vi "Main Config.vi"(8 "error in (no error)":errorcluster, 11 "Module_Refs":T1={"ModuleName"=enum."Controller", "Queue"=refnum, "user event"=refnum, "VI Refnum"=refnum, "ShowFP"=FALSE, "StatesTracking Enabled"=FALSE}) -> (0 "error out":errorcluster)   [LabVIEW 2021, in "Configuration.lvlib"]
doc: "Main Module Template of the architecture. Use this as a template to integrate new independent processes into your application."
uses:
  Configuration.lvlib
  Typedefs/Module References.ctl
  Typedefs/Enum_Module_Name.ctl
  Typedefs/Message.ctl
  Typedefs/SM Data.ctl
  Typedefs/App Cfg DVR.ctl
  Typedefs/Application Configuration.ctl
  Module Template/Typedefs/Config.ctl
  Core UI/Typedefs/Config.ctl
  Modules/Sound Manager/Typedefs/Config.ctl
  Typedefs/FGV Ref. Modules Function.ctl
  <vilib>/event_ctls.llb/usereventprio.ctl
  Architecture.lvlib
  Modules/Sound Manager/Sound Manager.lvlib
  Core UI/Core UI.lvlib
  Module Template/Module Template.lvlib
panel:
  in  "Stop App":bool
  out "Message":string
  in  "Stop Module":bool
  # "#Architecture\n\nPlace inside this box all visible data."
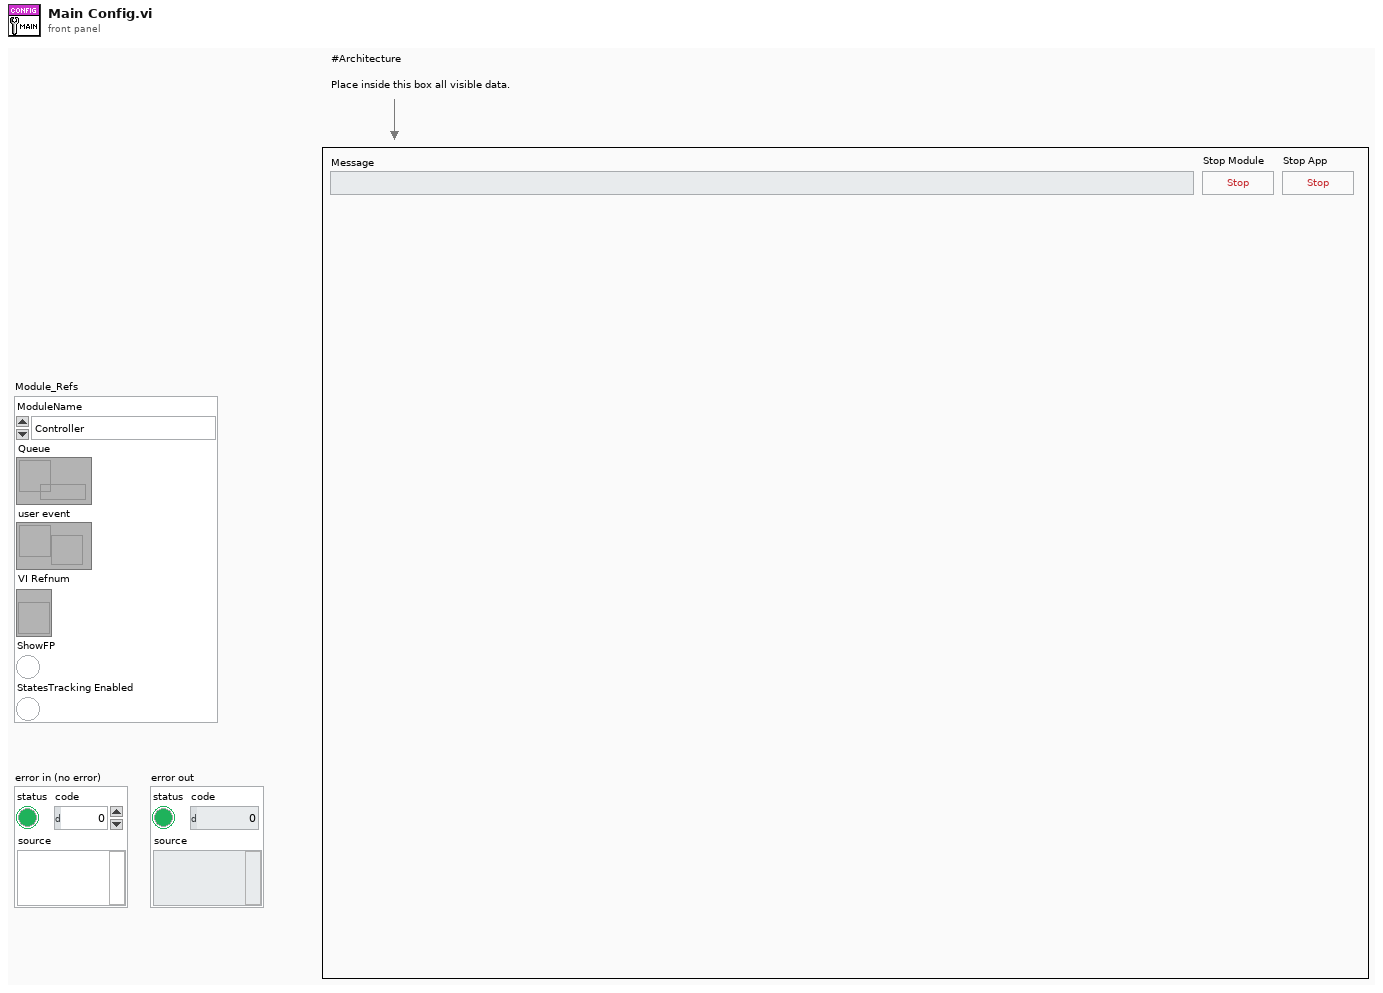
[diagram p1: front panel]
types:
  T1 = typedef "Architecture.lvlib/Module References.ctl" = cluster{"ModuleName":T2, "Queue":refnum<queue>, "user event":refnum<user-event>, "VI Refnum":refnum<vi>, "ShowFP":bool, "StatesTracking Enabled":bool}
  T2 = typedef "Configuration.lvlib/Enum_Module_Name.ctl" = enum16{"Configuration", "Error_Handler", "Log", "Database", "Controller", "UI Module", "Sound Manager"}
  T3 = typedef "Configuration.lvlib/SM Data.ctl" = cluster{"Module_Refs":T1, "Response Data":variant, "Config app":T4}
  T4 = typedef "Configuration.lvlib/App Cfg DVR.ctl" = refnum<data-value>
  T5 = enum32{"Invalid", "Standard", "Closed", "Hidden", "Minimized", "Maximized"}
  T6 = typedef "Error_Manager.lvlib/LogRotate.lvclass/LogData.ctl" = cluster{"error in":errorcluster, "replacements":string[], "Time Stamp":timestamp}
  T7 = typedef "Architecture.lvlib/FGV Ref. Modules Function.ctl" = enum16{"Init ", "Add Module", "Get Module", "Get All", "Add Asynchronous Run Ref", "Dispose"}
  T8 = typedef "usereventprio.ctl" = enum32{"high priority", "normal priority"}
  T9 = typedef "Configuration.lvlib/Application Configuration.ctl" = cluster{"Module Template Config":T10, "Core UI Config":T11, "Sound Manager Config":T12}
  T10 = typedef "Module Template.lvlib/Config.ctl" = cluster{"Module Enabled":bool}
  T11 = typedef "Core UI.lvlib/Config.ctl" = cluster{"Module Enabled":bool}
  T12 = typedef "Sound Manager.lvlib/Config.ctl" = cluster{"Sound Library Path":path, "dyn sounds path":path}
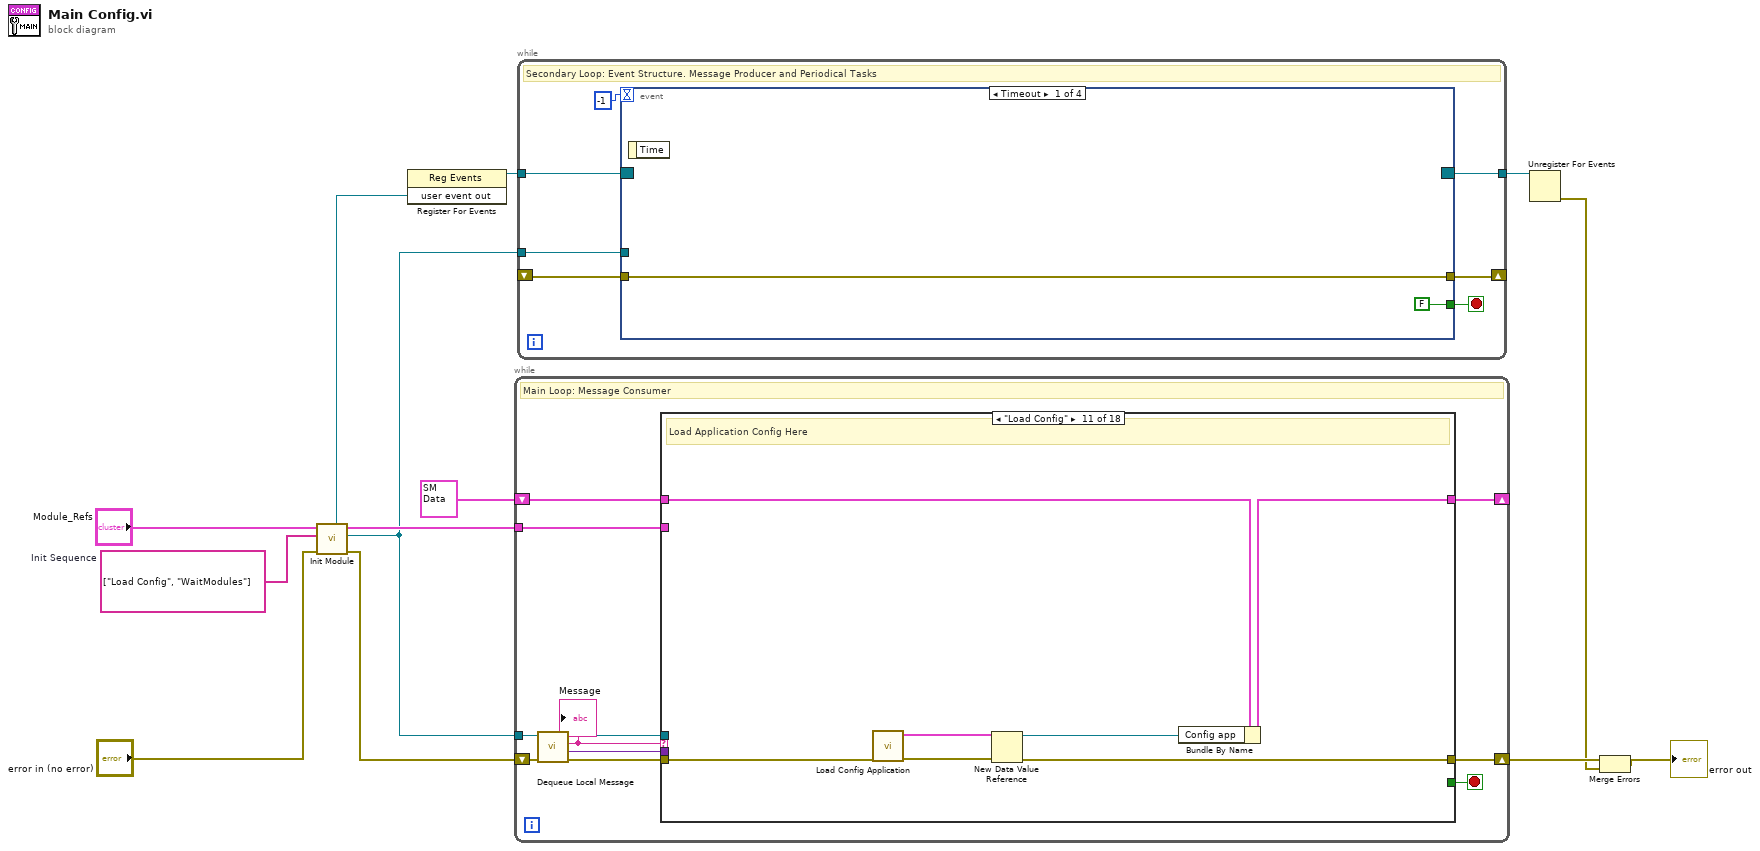
[diagram p0: block diagram]
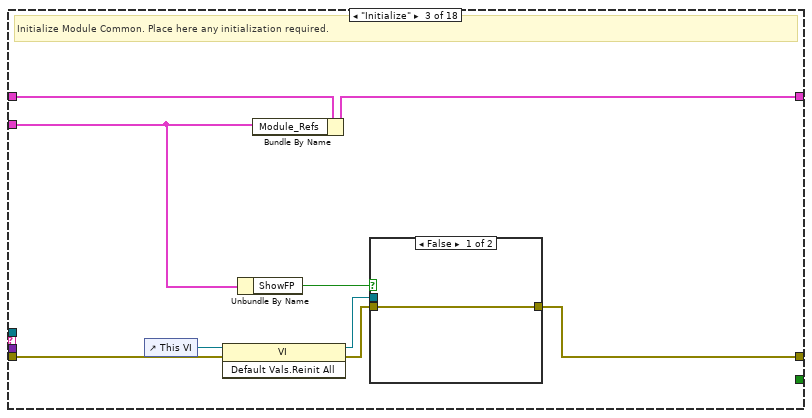
[diagram p4: hidden frame]
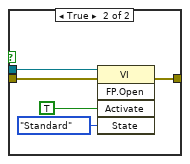
[diagram p5: hidden frame]
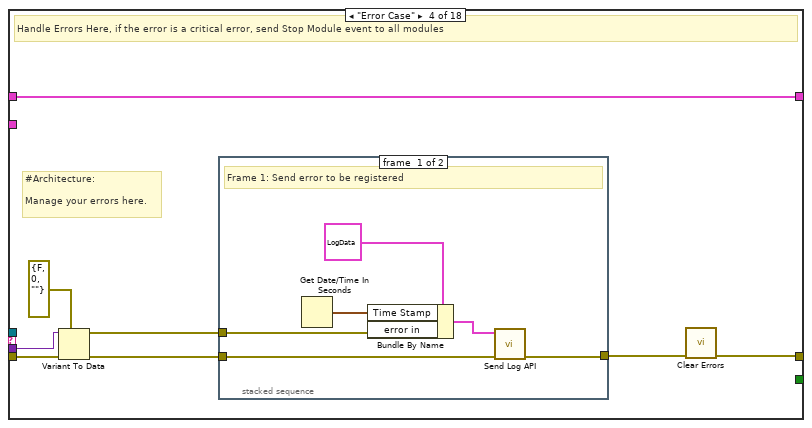
[diagram p6: hidden frame]
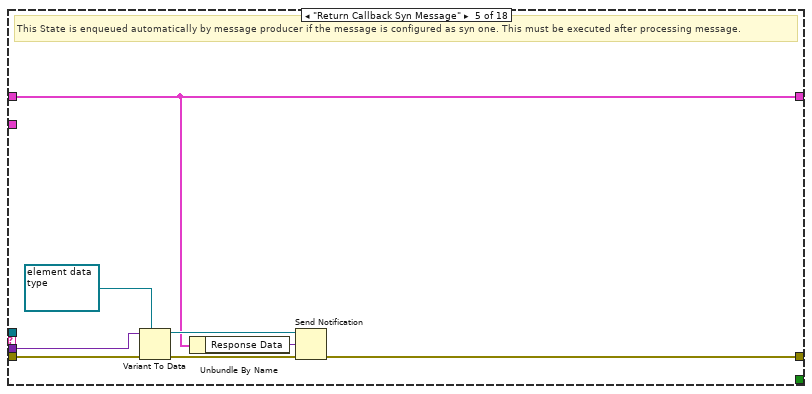
[diagram p9: hidden frame]
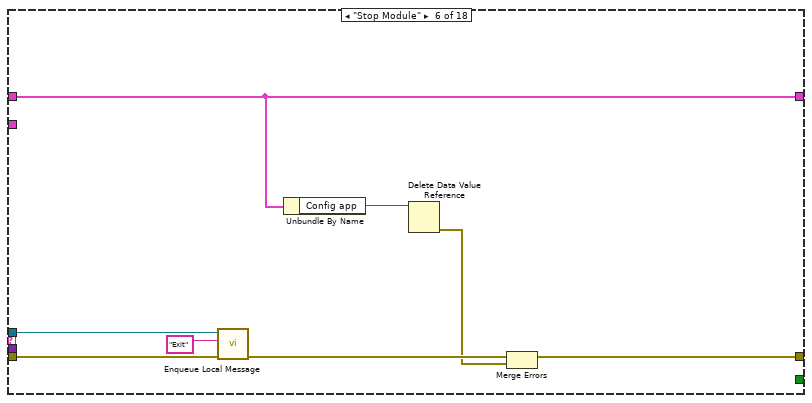
[diagram p10: hidden frame]
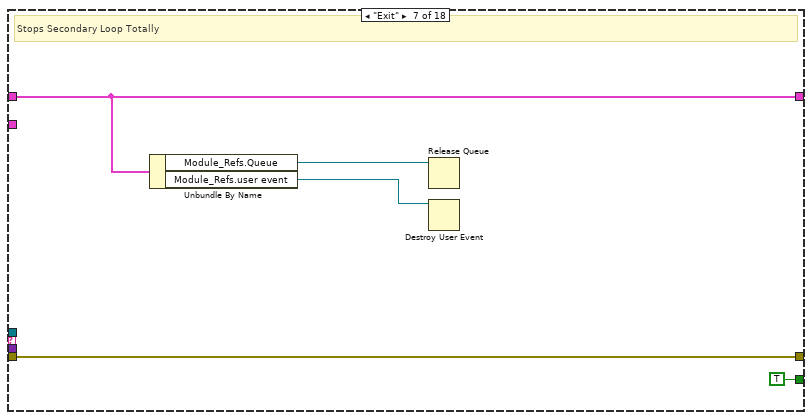
[diagram p11: hidden frame]
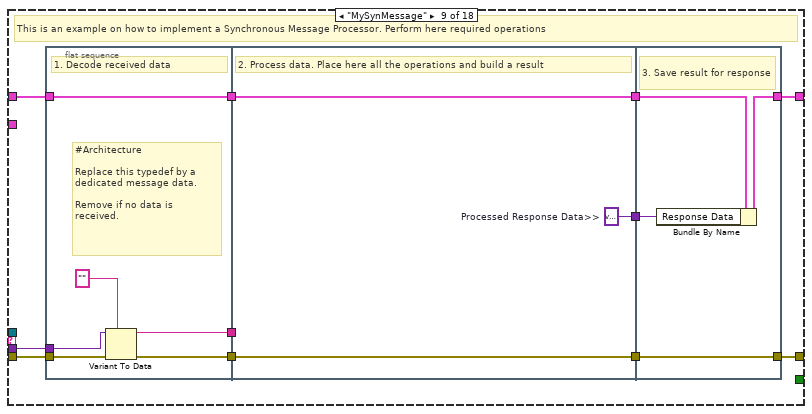
[diagram p13: hidden frame]
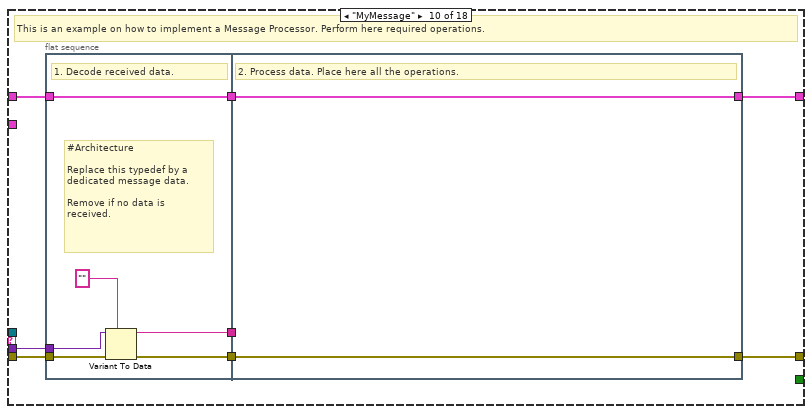
[diagram p14: hidden frame]
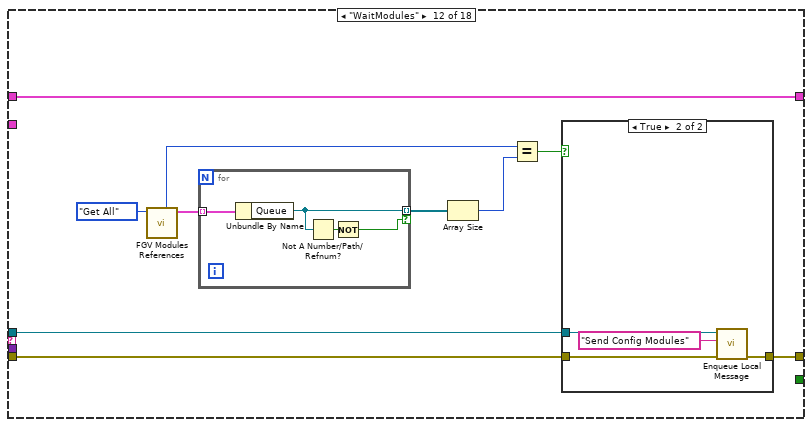
[diagram p15: hidden frame]
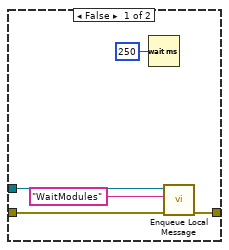
[diagram p16: hidden frame]
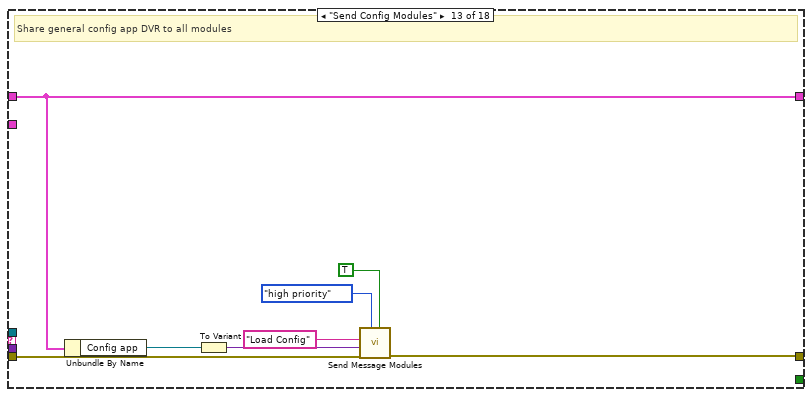
[diagram p17: hidden frame]
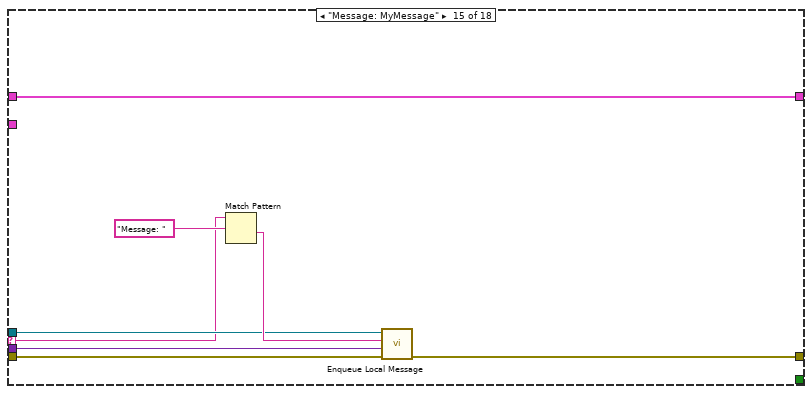
[diagram p19: hidden frame]
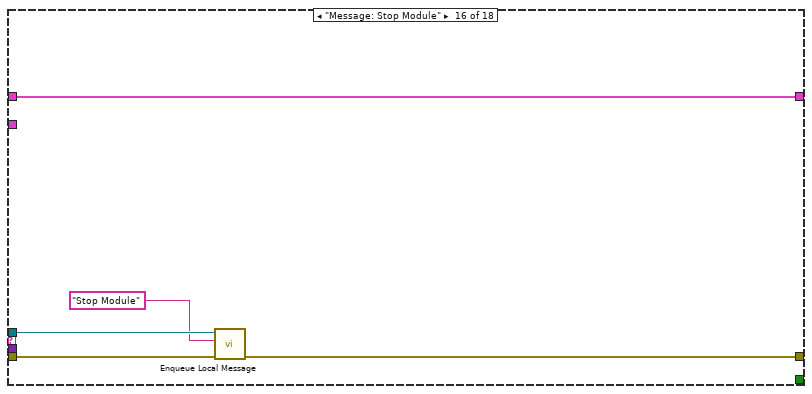
[diagram p20: hidden frame]
diagram:
  w11 = string[] ["Load Config", "WaitModules"]  # Init Sequence
  n1 = call "Init Module.vi"("error in (no error)"="error in (no error)", "Init Sequence"=w11, "Module Refs"="Module_Refs") -> ("error out"=w13:errorcluster, "queue out"=w2:refnum<queue>, "Module Refs Out"=w4:T1, "user event out"=w3:refnum<user-event>)  [unwired: 5 in]
  n2 = register-events(w3) -> (reference out=w10:refnum<event-registration>)  [unwired: 2 in, 1 out]
  n3 = while {
    shift-right: [w23] -> _
    shift-left: T3 {"Module_Refs"={"ModuleName"=enum."Controller", "Queue"=refnum, "user event"=refnum, "VI Refnum"=refnum, "ShowFP"=FALSE, "StatesTracking Enabled"=FALSE}, "Response Data"=variant, "Config app"=refnum} ("SM Data") -> [w24]
    shift-right: [w22] -> w8
    shift-left: w13 -> [w20]
    tunnel: w2 -> [w21]
    tunnel: w4 -> [w14]
    stop <- w15 stop-if-true
    # "Main Loop: Message Consumer"
    n4 = call "Dequeue Local Message.vi"("error in"=w20, "Msg queue in"=w21) -> ("error out"=w19:errorcluster, "Data"=w16:variant, "Message"=w17:string, "queue out"=w18:refnum<queue>)  [unwired: 6 in]
    "Message" <- w17
    n5 = case shown="\"Load Config\"" w17 {
      selector: w17 -> [_ _ _ _ _ _ _ _ _ _ _ _ _ _ w165 _ _ w188]
      tunnel: w24 -> [w26 w28 w37 w51 w63 w73 w80 w84 w95 w116 w131 w141 w157 w164 w172 w177 w179 w193]
      tunnel: [w26 w28 w35 w51 w63 w73 w80 w84 w94 w109 w127 w141 w157 w164 w172 w177 w179 w193] -> w23
      tunnel: w19 -> [w25 w27 w36 w50 w69 w77 w82 w83 w88 w112 w130 w134 w162 w163 w169 w176 w178 w192]
      tunnel: [w25 w27 w31 w44 w68 w72 w82 w83 w93 w115 w126 w133 w161 w163 w166 w175 w178 w182] -> w22
      tunnel: w18 -> [_ _ _ _ _ w75 _ _ _ _ _ w135 _ _ w167 w174 _ w189]
      tunnel: w16 -> [_ _ _ w49 w66 _ _ _ w87 w111 _ _ _ _ w168 _ _ w190]
      tunnel: [_ _ _ _ _ _ TRUE _ _ _ _ _ _ _ _ _ _ _] -> w15
      tunnel: w14 -> [_ _ w34 _ _ _ _ _ _ _ _ _ _ _ _ _ _ _]
      frame "--------State Machine Arquitechture Operations--------" {
      }
      frame "Idle", Default {
        # "Use this state to make iterations if required."
      }
      frame "Initialize" {
        # "Initialize Module Common. Place here any initialization required."
        n6 = control-ref of="This VI"() -> (w29:refnum<vi>)
        n7 = invoke class="VI" method="Default Vals.Reinit All"(reference=w29, error in=w36) -> (reference out=w32:refnum<vi>, error out=w33:errorcluster)  [unwired: 1 in, 1 out]
        n8 = Unbundle By Name(w34) -> ("ShowFP"=w30:bool)
        n9 = Bundle By Name(cluster=w37, "Module_Refs"=w34) -> (w35:T3)
        n10 = case shown="False" w30 {
          tunnel: w33 -> [w38 w43]
          tunnel: [w38 w42] -> w31
          tunnel: w32 -> [_ w41]
          frame False {
          }
          frame True {
            n11 = invoke class="VI" method="FP.Open"(reference=w41, error in=w43, "Activate"=TRUE ("Activate?"), "State"=T5."Standard") -> (error out=w42:errorcluster)  [unwired: 1 in, 4 out]
          }
        }
      }
      frame "Error Case" {
        # "#Architecture: \n\nManage your errors here."
        # "Handle Errors Here, if the error is a critical error, send Stop Module event to all modules"
        n12 = Variant To Data(error in=w50, type=errorcluster {"status"=FALSE, "code"=0, "source"=""} ("error constant"), Variant=w49) -> (data=w45:errorcluster, error out=w47:errorcluster)
        n13 = stacked-sequence {
          tunnel: w47 -> [w57 w59]
          tunnel: [w56 _] -> w46
          tunnel: w45 -> [w54 w58]
          frame #0 {
            # "Frame 1: Send error to be registered"
            n14 = Get Date/Time In Seconds() -> (seconds since 1Jan1904=w53:timestamp)
            n15 = Bundle By Name(cluster=T6 {"error in"={"status"=FALSE, "code"=0, "source"=""}, "replacements"=[], "Time Stamp"=timestamp(0 s since 1904-01-01)} ("Data"), "Time Stamp"=w53, "error in"=w54) -> (w52:T6)
            n16 = call "Send Log API.vi"("error in (no error)"=w57, "Data"=w52) -> ("error out"=w56:errorcluster)  [unwired: 9 in]
          }
          frame #1 {
            # "Frame 2: Manage your errors here"
            n17 = case shown="No Error" w58 {
              tunnel: [w60 w61] -> _
              tunnel: w59 -> [w60 w61]
              frame No Error {
              }
              frame Error {
                # "#Architecture \n\nPlace here critical errors to be managed \nin the desired way."
              }
            }
          }
        }
        n18 = call <vilib>:"Clear Errors.vi"("error in (no error)"=w46) -> ("error out"=w44:errorcluster)  [unwired: 5 in, 1 out]
      }
      frame "Return Callback Syn Message" {
        # "This State is enqueued automatically by message producer if the message is configured as syn one. This must be executed after processing message."
        n19 = Variant To Data(error in=w69, type=refnum<notifier> refnum ("notifier out"), Variant=w66) -> (data=w64:refnum<notifier>, error out=w67:errorcluster)
        n20 = Unbundle By Name(w63) -> ("Response Data"=w62:variant)
        n21 = Send Notification(notification=w62, notifier=w64, error in (no error)=w67) -> (error out=w68:errorcluster)  [unwired: 1 out]
      }
      frame "Stop Module" {
        n22 = call "Enqueue Local Message.vi"("error in"=w77, "Message"="Exit", "Msg queue in"=w75) -> ("error out"=w76:errorcluster)  [unwired: 7 in, 1 out]
        n23 = Unbundle By Name(w73) -> ("Config app"=w71:T4)
        n24 = Delete Data Value Reference(data value reference=w71) -> (error out=w70:errorcluster)  [unwired: 1 in, 1 out]
        n25 = Merge Errors(w76, w70) -> (w72:errorcluster)
      }
      frame "Exit" {
        # "Stops Secondary Loop Totally"
        n26 = Unbundle By Name(w80) -> ("Module_Refs.Queue"=w79:refnum<queue>, "Module_Refs.user event"=w78:refnum<user-event>)
        n27 = Release Queue(queue=w79) -> ()  [unwired: 2 in, 3 out]
        n28 = Destroy User Event(user event=w78) -> ()  [unwired: 1 in, 1 out]
      }
      frame "--------------State Machine Custom States-------------" {
      }
      frame "MySynMessage" {
        # "This is an example on how to implement a Synchronous Message Processor. Perform here required operations"
        n29 = flat-sequence {
          tunnel: w88 -> [w99]
          tunnel: w95 -> [w101]
          tunnel: [w101] -> w92
          tunnel: [w97] -> w91
          tunnel: w87 -> [w98]
          tunnel: [w96] -> w86
          tunnel: w92 -> [w104]
          tunnel: w91 -> [w103]
          tunnel: [w104] -> w90
          tunnel: [w103] -> w89
          tunnel: w86 -> [_]
          tunnel: [w102] -> w85
          tunnel: [w107] -> w93
          tunnel: [w106] -> w94
          tunnel: w90 -> [w108]
          tunnel: w89 -> [w107]
          tunnel: w85 -> [w105]
          frame #0 {
            # "#Architecture\n\nReplace this typedef by a dedicated message data.\n\nRemove if no data is received."
            # "1. Decode received data"
            n30 = Variant To Data(error in=w99, type="", Variant=w98) -> (data=w96:string, error out=w97:errorcluster)
          }
          frame #1 {
            w102 = variant  # Processed Response Data>>
            # "2. Process data. Place here all the operations and build a result"
          }
          frame #2 {
            # "3. Save result for response"
            n31 = Bundle By Name(cluster=w108, "Response Data"=w105) -> (w106:T3)
          }
        }
      }
      frame "MyMessage" {
        # "This is an example on how to implement a Message Processor. Perform here required operations."
        n32 = flat-sequence {
          tunnel: w112 -> [w120]
          tunnel: w116 -> [w122]
          tunnel: [w122] -> w114
          tunnel: [w118] -> w113
          tunnel: w111 -> [w119]
          tunnel: [w117] -> w110
          tunnel: w114 -> [w123]
          tunnel: w113 -> [w124]
          tunnel: w110 -> [_]
          tunnel: [w124] -> w115
          tunnel: [w123] -> w109
          frame #0 {
            # "#Architecture\n\nReplace this typedef by a dedicated message data.\n\nRemove if no data is received."
            # "1. Decode received data."
            n33 = Variant To Data(error in=w120, type="", Variant=w119) -> (data=w117:string, error out=w118:errorcluster)
          }
          frame #1 {
            # "2. Process data. Place here all the operations."
          }
        }
      }
      frame "Load Config" {
        # "Load Application Config Here"
        n34 = call "Load Config Application.vi"("error In"=w130) -> ("error Out"=w129:errorcluster, "Application Configuration"=w128:T9)  [unwired: 9 in]
        n35 = New Data Value Reference(data value=w128, error in=w129) -> (data value reference=w125:refnum<data-value>, error out=w126:errorcluster)
        n36 = Bundle By Name(cluster=w131, "Config app"=w125) -> (w127:T3)
      }
      frame "WaitModules" {
        n37 = call "FGV Modules References.vi"("FGV Ref. Function In"=FGV_Ref._Modules_Function."Get All") -> ("All Modules Refs"=w139:T1[], "size out"=w136:i32)  [unwired: 7 in, 2 out]
        n38 = for {
          tunnel: w139 -> [w154] mode=indexing
          tunnel: [w153] -> w138 mode=indexing if=w151
          n39 = Unbundle By Name(w154) -> ("Queue"=w153:refnum<queue>)
          n40 = Not A Number/Path/Refnum?(number/path/refnum=w153) -> (NaN/Path/Refnum?=w152:bool)
          n41 = Not(x=w152) -> (.not. x?=w151:bool)
        }
        n42 = Array Size(array=w138) -> (size(s)=w137:i32)
        n43 = Equal?(x=w136, y=w137) -> (x = y?=w132:bool)
        n44 = case shown="True" w132 {
          tunnel: w135 -> [w144 w148]
          tunnel: w134 -> [w146 w150]
          tunnel: [w145 w149] -> w133
          frame False {
            n45 = Wait (ms)(milliseconds to wait=u32 250) -> ()  [unwired: 1 out]
            n46 = call "Enqueue Local Message.vi"("error in"=w146, "Message"="WaitModules", "Msg queue in"=w144) -> ("error out"=w145:errorcluster)  [unwired: 7 in, 1 out]
          }
          frame True {
            n47 = call "Enqueue Local Message.vi"("error in"=w150, "Message"="Send Config Modules", "Msg queue in"=w148) -> ("error out"=w149:errorcluster)  [unwired: 7 in, 1 out]
          }
        }
      }
      frame "Send Config Modules" {
        # "Share general config app DVR to all modules"
        n48 = Unbundle By Name(w157) -> ("Config app"=w156:T4)
        n49 = To Variant(anything=w156) -> (Variant=w155:variant)
        n50 = call "Send Message Modules.vi"("All Modules"=TRUE, "priority (normal)"=usereventprio."high priority", "Error In"=w162, "Data"=w155, "Message"="Load Config") -> ("error in (no error)"=w161:errorcluster)  [unwired: 6 in]
      }
      frame "--------------Dynamic Events Messages----------------" {
      }
      frame "Message: MyMessage" {
        n51 = Match Pattern(string=w165, regular expression="Message: ") -> (after substring=w170:string)  [unwired: 1 in, 3 out]
        n52 = call "Enqueue Local Message.vi"("error in"=w169, "Data"=w168, "Message"=w170, "Msg queue in"=w167) -> ("error out"=w166:errorcluster)  [unwired: 6 in, 1 out]
      }
      frame "Message: Stop Module" {
        n53 = call "Enqueue Local Message.vi"("error in"=w176, "Message"="Stop Module", "Msg queue in"=w174) -> ("error out"=w175:errorcluster)  [unwired: 7 in, 1 out]
      }
      frame "------------Synchronous Event Messages--------------" {
      }
      frame "SynMessage: MySynMessage" {
        # "Use this case as a handler for Synchronous messages. This state queues a message for the desired"
        n54 = call "Extract Synchronous Data.vi"("error in 2"=w192, "Variant"=w190) -> ("error in"=w191:errorcluster, "Data Out"=w185:variant, "notifier out"=w180:refnum<notifier>)  [unwired: 7 in]
        n55 = Match Pattern(string=w188, regular expression="SynMessage: ") -> (after substring=w186:string)  [unwired: 1 in, 3 out]
        n56 = call "Enqueue Local Message.vi"("error in"=w191, "Data"=w185, "Message"=w186, "Msg queue in"=w189) -> ("error out"=w184:errorcluster, "queue out"=w183:refnum<queue>)  [unwired: 6 in]
        n57 = call "Enqueue Local Message.vi"("error in"=w184, "Data"=w180, "Message"="Return Callback Syn Message", "Msg queue in"=w183) -> ("error out"=w182:errorcluster)  [unwired: 6 in, 1 out]
      }
    }
  }
  n58 = while {
    tunnel: w10 -> [w200]
    tunnel: w2 -> [w197]
    tunnel: [w196] -> w9
    shift-right: [w194] -> _
    shift-left: _ -> [w195]
    stop <- w198 stop-if-true
    # "Secondary Loop: Event Structure. Message Producer and Periodical Tasks"
    n59 = event shown="[0] Timeout" {
      selector: w200 -> [_ _ _ _]
      dyn-events: [_ _ _ _] -> w196
      timeout: -1 -> [_ _ _ _]
      tunnel: [FALSE w209 TRUE _] -> w198
      tunnel: w197 -> [_ w214 w216 _]
      tunnel: w195 -> [w201 w213 w219 w221]
      tunnel: [w201 w212 w217 w220] -> w194
      event Timeout {
        n60 = event-data() -> ()  [unwired: 1 in, 1 out]
      }
      event User Event {
        # "Send message to local queue. \n(Message Consumer)"
        # "Processes an external event and enqueues a message to the local queue. It can be synchronous (with response) or NOT."
        n61 = event-data() -> ("syn"=w206:bool, "Message"=w208:string, "Data"=w211:variant)  [unwired: 1 in]
        n62 = Select(t="SynMessage: " ("string"), s=w206, f="Message: " ("string")) -> (s? t:f=w203:string)
        n63 = Concatenate Strings(w203, w208) -> (w210:string)
        n64 = call "Enqueue Local Message.vi"("error in"=w213, "Data"=w211, "Message"=w210, "Msg queue in"=w214) -> ("error out"=w212:errorcluster)  [unwired: 6 in, 1 out]
        n65 = Equal?(x=w208, y="Stop Module") -> (x = y?=w209:bool)
      }
      event "Stop Module": Value Change {
        n66 = event-data() -> ()  [unwired: 1 in, 1 out]
        n67 = call "Enqueue Local Message.vi"("error in"=w219, "Message"="Stop Module", "Msg queue in"=w216) -> ("error out"=w217:errorcluster)  [unwired: 7 in, 1 out]
      }
      event "Stop App": Value Change {
        w223 = TRUE  # All Modules
        # "Send Stop To All Modules"
        n68 = event-data() -> ()  [unwired: 1 in, 1 out]
        n69 = call "Send Message Modules.vi"("All Modules"=w223, "Error In"=w221, "Message"="Stop Module") -> ("error in (no error)"=w220:errorcluster)  [unwired: 8 in]
      }
    }
  }
  n70 = Unregister For Events(event registration refnum=w9) -> (error out=w7:errorcluster)  [unwired: 1 in]
  n71 = Merge Errors(w8, w7) -> (→"error out":errorcluster)
